vi "Sequence Templetdata inquiry.vi"(0 "VISA resource name":refnum<visa-resource-name>, 1 "Channel  (1: CH1)":u16(ring)=1 items=["CH1"=1, "CH2"=2, "CH3"=3, "CH4"=4], 11 "error in (no error)":errorcluster) -> (2 "Object":string, 3 "Type":string, 4 "VISA resource name out":refnum<visa-resource-name>, 6 "MAX Value":dbl, 8 "MIN Value":dbl, 10 "Start":dbl, 12 "Inverted":string, 13 "Interval":dbl, 14 "Points":dbl, 15 "error out":errorcluster)   [LabVIEW 2020, in "GPP.lvlib"]
uses:
  GPP.lvlib
  Function/VISA_COMMON.ctl
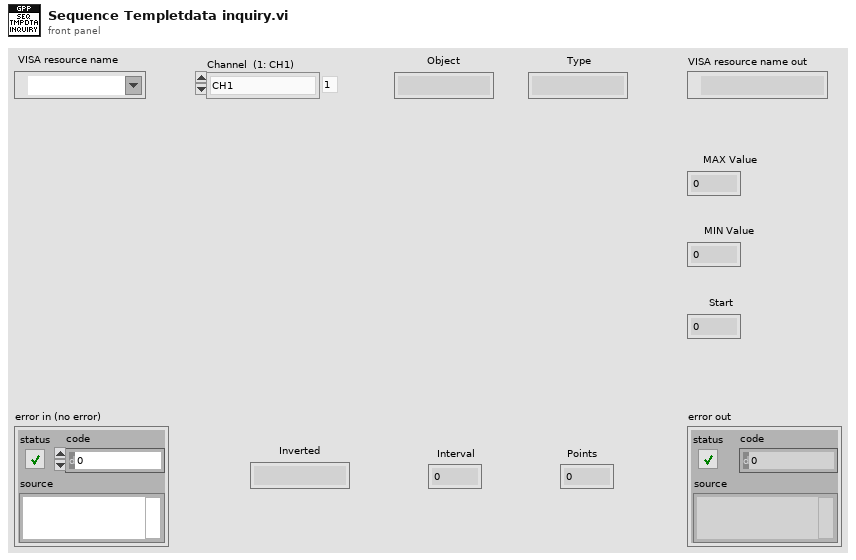
[diagram p1: front panel]
types:
  T1 = typedef "GPP.lvlib/VISA_COMMON.ctl" = enum16{"Initial", "Write CMD", "Read Result", "Read History", "Close"}
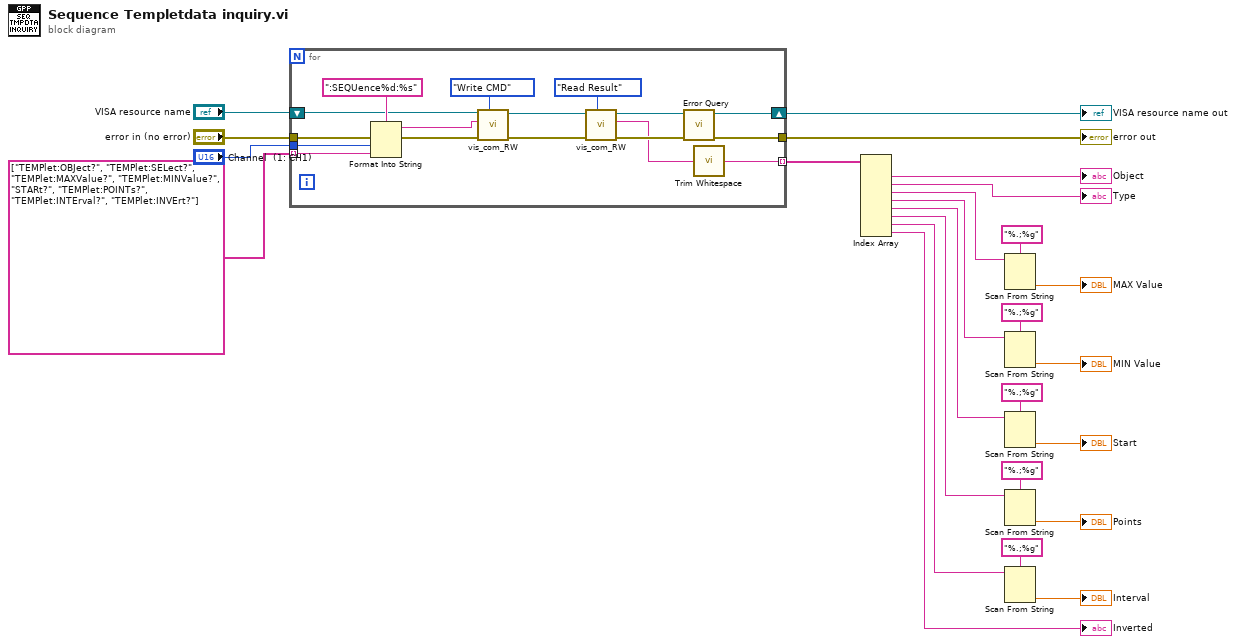
[diagram p0: block diagram]
diagram:
  n1 = for {
    tunnel: "error in (no error)" -> [w36]
    tunnel: "Channel  (1: CH1)" -> [w34]
    tunnel: string[] ["TEMPlet:OBJect?", "TEMPlet:SELect?", "TEMPlet:MAXValue?", "TEMPlet:MINValue?", "STARt?", "TEMPlet:POINTs?", "TEMPlet:INTErval?", "TEMPlet:INVErt?"] -> [w31] mode=indexing
    tunnel: [w32] -> w18
    tunnel: [w28] -> w22 mode=indexing
    shift-right: [w26] -> w17
    shift-left: "VISA resource name" -> [w30]
    n2 = Format Into String(format string=":SEQUence%d:%s", error in=w36, w34, w31) -> (resulting string=w29:string, error out=w35:errorcluster)  [unwired: 1 in]
    n3 = call "vis_com_RW.vi"("Funciton"=VISA_COMMON."Write CMD", "error in (no error)"=w35, "CMD String"=w29, "VISA resource in"=w30) -> ("error out"=w40:errorcluster, "VISA resource out"=w39:refnum<visa-resource-name>)  [unwired: 5 in, 1 out]
    n4 = call "vis_com_RW.vi"("Funciton"=VISA_COMMON."Read Result", "error in (no error)"=w40, "VISA resource in"=w39) -> ("error out"=w37:errorcluster, "Result"=w27:string, "VISA resource out"=w38:refnum<visa-resource-name>)  [unwired: 6 in]
    n5 = call "Error Query.vi"("error in (no error)"=w37, "VISA resource name"=w38) -> ("error out"=w32:errorcluster, "VISA resource name out"=w26:refnum<visa-resource-name>)  [unwired: 6 in, 2 out]
    n6 = call <vilib>:"Trim Whitespace.vi"("string"=w27) -> ("trimmed string"=w28:string)  [unwired: 1 in]
  }
  "error out" <- w18
  "VISA resource name out" <- w17
  n7 = Index Array(array=w22) -> (element #1=→"Object":string, element #2=→"Type":string, element #3=w20:string, element #4=w10:string, element #5=w9:string, element #6=w8:string, element #7=w7:string, element #8=→"Inverted":string)  [unwired: 8 in]
  n8 = Scan From String(format string="%.;%g", input string=w20) -> (output 1=→"MAX Value":dbl)  [unwired: 3 in, 3 out]
  n9 = Scan From String(format string="%.;%g", input string=w10) -> (output 1=→"MIN Value":dbl)  [unwired: 3 in, 3 out]
  n10 = Scan From String(format string="%.;%g", input string=w9) -> (output 1=→"Start":dbl)  [unwired: 3 in, 3 out]
  n11 = Scan From String(format string="%.;%g", input string=w8) -> (output 1=→"Points":dbl)  [unwired: 3 in, 3 out]
  n12 = Scan From String(format string="%.;%g", input string=w7) -> (output 1=→"Interval":dbl)  [unwired: 3 in, 3 out]
